vi "Choose_File_Type.vi"(8 "error in (no error)":errorcluster) -> (0 "error out":errorcluster, 2 "OK?":bool, 3 "File Type Out":T1)   [LabVIEW 2024]
uses:
  controls/file_type.ctl
panel:
  in  "File Type":T1
  in  "Cancel":bool
  in  "OK":bool
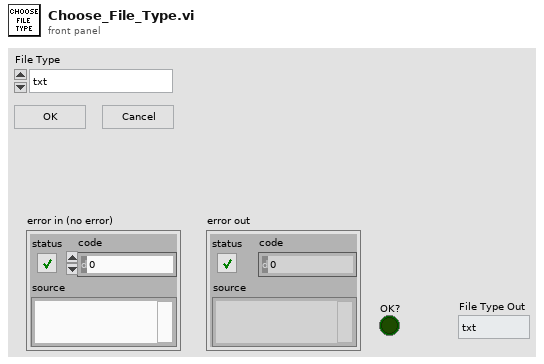
[diagram p1: front panel]
types:
  T1 = typedef "file_type.ctl" = enum16{"txt", "csv", "tdms"}
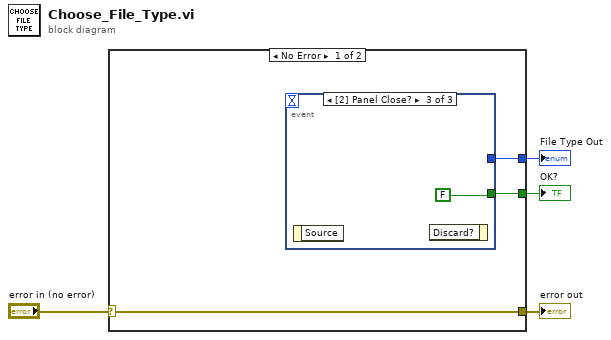
[diagram p0: block diagram]
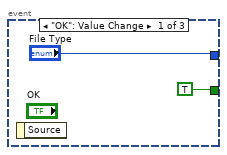
[diagram p2: hidden frame]
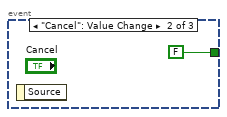
[diagram p3: hidden frame]
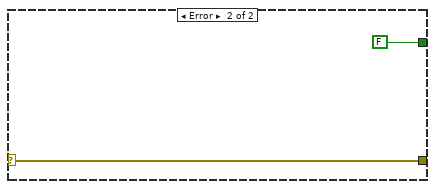
[diagram p4: hidden frame]
diagram:
  n1 = case shown="No Error" "error in (no error)" {
    selector: "error in (no error)" -> [w7 w13]
    tunnel: [w7 w13] -> w3
    tunnel: [w6 _] -> w2
    tunnel: [w5 FALSE] -> w1
    frame No Error {
      n2 = event shown="[2] Panel Close?" {
        selector: _ -> [_ _ _]
        dyn-events: _ -> [_ _ _]
        timeout: _ -> [_ _ _]
        tunnel: ["File Type" _ _] -> w6
        tunnel: [TRUE FALSE FALSE] -> w5
        event "OK": Value Change {
          n3 = event-data() -> ()  [unwired: 1 in, 1 out]
        }
        event "Cancel": Value Change {
          n4 = event-data() -> ()  [unwired: 1 in, 1 out]
        }
        event Panel Close? {
          n5 = event-data() -> ()  [unwired: 1 in, 1 out]
          n6 = event-data() -> ()  [unwired: 2 in, 1 out]
        }
      }
    }
    frame Error {
    }
  }
  "error out" <- w3
  "File Type Out" <- w2
  "OK?" <- w1
